vi "Save_to_Project.vi"(8 "error in (no error)":errorcluster, 9 "index":i32, 10 "Item Ref":T1, 11 "AB_Source_Exported_Assembly_VI in":refnum<class "AB_Source_Exported_Assembly_VI.lvclass">) -> (0 "error out":errorcluster, 3 "AB_Source_Exported_Assembly_VI out":refnum<class "AB_Source_Exported_Assembly_VI.lvclass">)   [LabVIEW 2020, in "AB_Source_Exported_Assembly_VI.lvclass"]
uses:
  <vilib>/AppBuilder/AB_Classes/Source/ExportedAssemblyVI/AB_Source_Exported_Assembly_VI.lvclass
  <resource>/Framework/Providers/API/ItemRef.ctl
  <vilib>/AppBuilder/RW_Project/AB_RW_Project_Source_ExportedAssemblyVI_Data.ctl
  <vilib>/AppBuilder/AB_InteropAssembly_DistVI_Proto_Info.ctl
  <vilib>/AppBuilder/IOStatus.ctl
  <vilib>/AppBuilder/RW_Project/AB_RW_Project_PropBag_Action.ctl
  <vilib>/AppBuilder/AB_Classes/Source/ExportedAssemblyVI/AB_Source_Exported_Assembly_VI.lvclass/AB_Source_Exported_Assembly_VI.ctl
  <vilib>/AppBuilder/AB_Classes/Source/VI/AB_Source_VI.lvclass
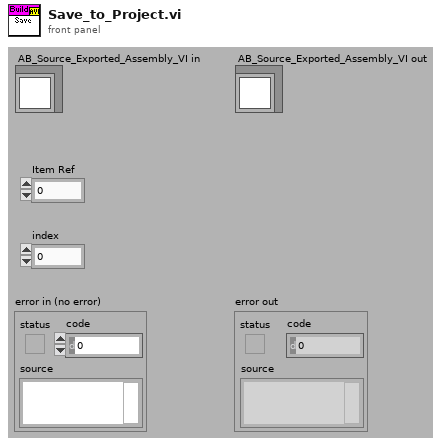
[diagram p1: front panel]
types:
  T1 = typedef "ItemRef.ctl" = u64
  T2 = typedef "AB_RW_Project_Source_ExportedAssemblyVI_Data.ctl" = cluster{"ExportAssemblyVIinfo":T3}
  T3 = typedef "AB_InteropAssembly_DistVI_Proto_Info.ctl" = cluster{"Library Name":string, "VI Name":string, "Method Name":string, "LV Class":path, "Param Names":string[], "Data Types":string[], "Dirs":T4[], "InputIdx":i32[], "OutputIdx":i32[], "ConNum":i8[], "IsCustomDocumentation":bool, "Custom Documentation":string, "IsProtected":bool, "IsSanitized":bool}
  T4 = typedef "IOStatus.ctl" = enum16{"Input", "Output", "Input/Output", "InputDeleted", "OutputDeleted", "IODeleted", "ErrorClusterIn", "ErrorClusterOut"}
  T5 = typedef "AB_RW_Project_PropBag_Action.ctl" = enum16{"read", "write", "clear", "readPrevious", "writePrevious", "clearPrevious"}
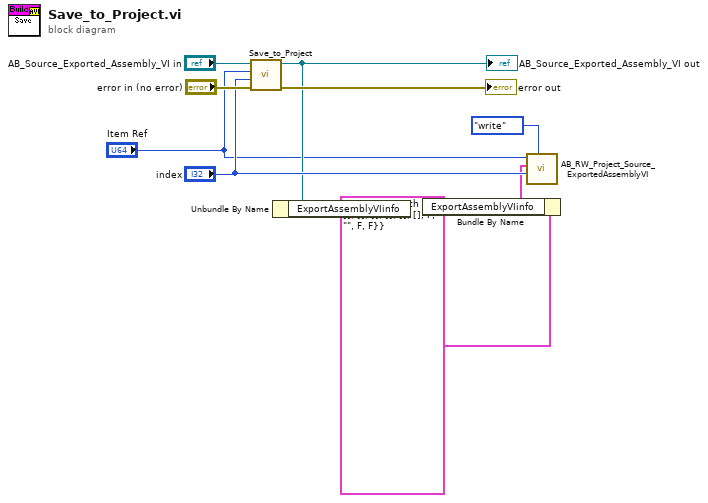
[diagram p0: block diagram]
diagram:
  n1 = call-parent "Save_to_Project.vi"("error in (no error)"="error in (no error)", "index"="index", "buildObject"="Item Ref", "AB_Source_VI in"="AB_Source_Exported_Assembly_VI in") -> ("error out"=→"error out":errorcluster, "AB_Source_VI out"=w5:refnum<class "AB_Source_Exported_Assembly_VI.lvclass">)  [unwired: 6 out]
  "AB_Source_Exported_Assembly_VI out" <- w5
  n2 = Unbundle By Name(w5) -> ("ExportAssemblyVIinfo"=w3:T3)
  n3 = Bundle By Name(cluster=T2 {"ExportAssemblyVIinfo"={"Library Name"="", "VI Name"="", "Method Name"="", "LV Class"=path "", "Param Names"=[], "Data Types"=[], "Dirs"=[], "InputIdx"=[], "OutputIdx"=[], "ConNum"=[], "IsCustomDocumentation"=FALSE, "Custom Documentation"="", "IsProtected"=FALSE, "IsSanitized"=FALSE}} ("dataSource in"), "ExportAssemblyVIinfo"=w3) -> (w4:T2)
  n4 = call <vilib>:"AB_RW_Project_Source_ExportedAssemblyVI.vi"("action"=AB_RW_Project_PropBag_Action."write", "index in"="index", "dataSource in"=w4, "buildObject"="Item Ref") -> ()  [unwired: 1 in, 7 out]
